vi "CT_IGPressureCheck.vi"(1 "IG1 Threshold":dbl=1e-06 format="%#_2e", 2 "Vacuum Sensors":T1={"IG1 On"=TRUE, "IG2On"=FALSE, "IG Vac Level"=7.206095277894153e-07, "CG1 Vac Level"=7.188197481794052e-05, "CG2 Vac Level"=7.698533430214743e-05, "IG Status"=TRUE, "Turbo Gate"=FALSE} {"CG2 Vac Level" format="%#_2e"; "CG1 Vac Level" format="%#_2e"; "IG Vac Level" format="%#_2e"}) -> (0 "IG Pressure Good":bool)   [LabVIEW 2016]
uses:
  VacuumControls.ctl
panel:
  out "Vacuum Sensors":T2={"TP On"=FALSE, "IG1 On"=FALSE, "IG2 On"=FALSE, "Cryo Pump"=FALSE, "IG Vac Level"=1.8050947371315723e-12, "CG1 Vac Level"=7.188197481794052e-05, "CG2 Vac Level"=7.628339269500514e-05} {"CG2 Vac Level" format="%#_2e"; "CG1 Vac Level" format="%#_2e"; "IG Vac Level" format="%#_2e"}
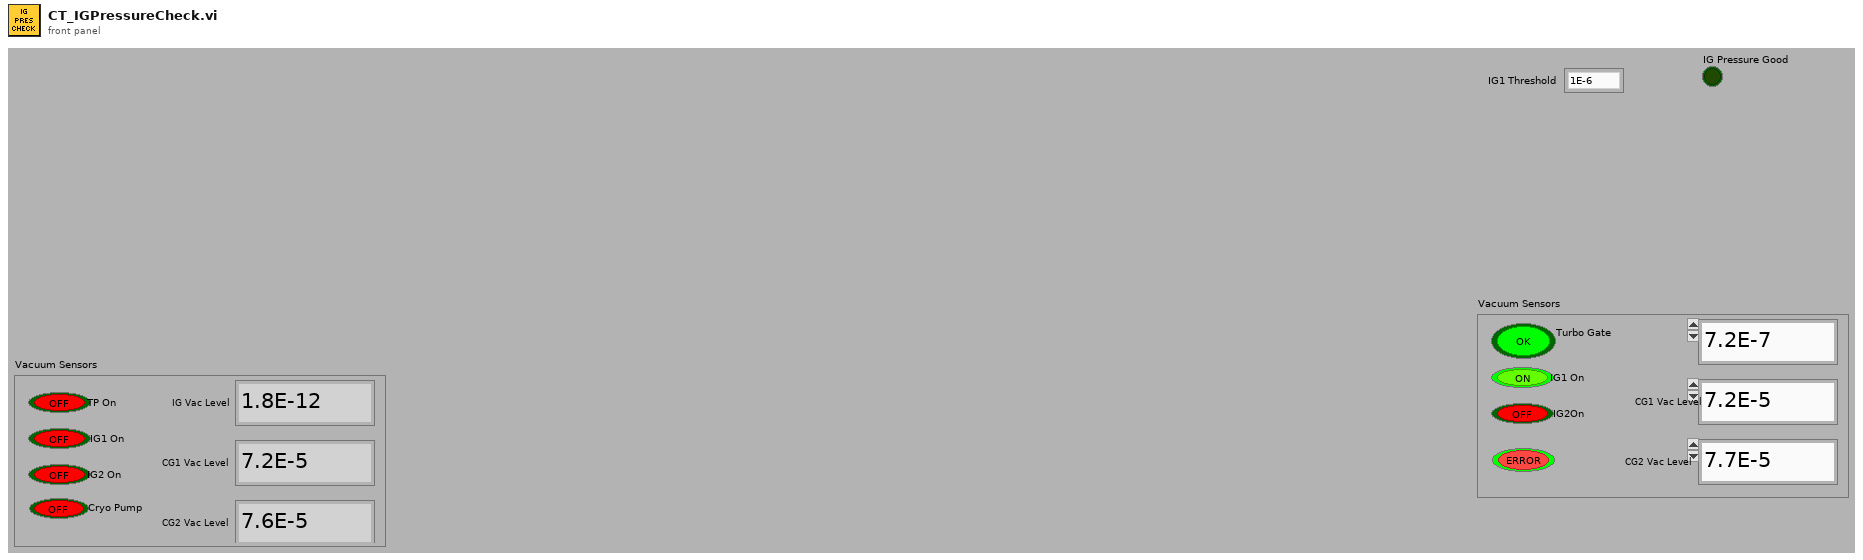
[diagram p1: front panel]
types:
  T1 = typedef "VacuumControls.ctl" = cluster{"IG1 On":bool, "IG2On":bool, "IG Vac Level":dbl, "CG1 Vac Level":dbl, "CG2 Vac Level":dbl, "IG Status":bool, "Turbo Gate":bool}
  T2 = cluster{"TP On":bool, "IG1 On":bool, "IG2 On":bool, "Cryo Pump":bool, "IG Vac Level":dbl, "CG1 Vac Level":dbl, "CG2 Vac Level":dbl}
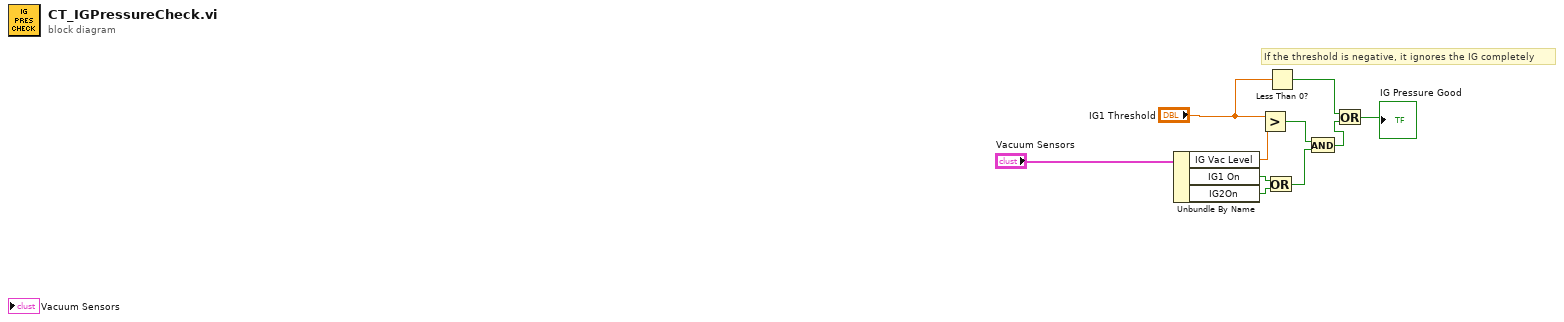
[diagram p0: block diagram]
diagram:
  # "If the threshold is negative, it ignores the IG completely"
  n1 = Unbundle By Name("Vacuum Sensors") -> ("IG Vac Level"=w10:dbl, "IG1 On"=w3:bool, "IG2On"=w2:bool)
  n2 = Greater?(x="IG1 Threshold", y=w10) -> (0:w8:bool)
  n3 = Or(x=w3, y=w2) -> (x .or. y?=w1:bool)
  n4 = Less Than 0?(x="IG1 Threshold") -> (x < 0?=w6:bool)
  n5 = And(x=w8, y=w1) -> (x .and. y?=w5:bool)
  n6 = Or(x=w6, y=w5) -> (x .or. y?=→"IG Pressure Good":bool)
